vi "Measurement UI.vi"() -> ()   [LabVIEW 2023, in "FPT Pulse Measurement UI.lvlib"]
uses:
  FPT Pulse Measurement UI.lvlib
panel:
  in  "Measurement Graph":T1(tab)
  out "General Graph 1":T2(graph)
  out "General Graph 2":T2(graph)
  out "General Graph 3":T2(graph)
  in  "Power sequencing file validity check":bool
  out "TS Acquired Amplitude":dbl[][](array[numeric])
  out "Per Pulse Result (Name)":string[](array[string])
  out "Phase Stability (dB)":dbl
  out "Amplitude Stability (dB)":dbl
  out "Overshoot (%)":dbl
  out "Ripple (%)":dbl
  out "Droop (%)":dbl
  out "Fall Time (us)":dbl
  out "Rising Time (us)":dbl
  out "Duty Cycle (%)":dbl
  out "Per Pulse Result":dbl[][](array[numeric])
  in  "Power sequencing file path":string
  in  "RFSG name":string="5842_0"
  in  "RFSG attenuation mode":T3(ring)=enum."s2p File"
  in  "RFSG s2p file path":string
  in  "RFmx name":string="5842_0"
  in  "RFmx attenuation mode":T3(ring)=enum."s2p File"
  in  "RFmx s2p file path":string
  out "All graph references":refnum<vi>[](array[refnum])
  out "TS P2P Stability":dbl[][](array[numeric])
  out "TS Intrapulse Stability":dbl[][](array[numeric])
  out "MeasTable":string[][](table)
  out "MeasTable 2":string[][](table)
  in  "Configuration":T4(ring)
  in  "Tab Control":T5(tab)
  in  "Power sequencing file":path caption="Power Sequencing File Path"
  in  "RFmx port":string(combo)="port2" caption="RFmx Port"
  in  "RFSG port":string(combo)="port1" caption="RFSG Port"
  in  "RFSG name_update":refnum<k15> caption="RFSG Name"
  in  "RFSG attenuation mode_tab":T3(tab)=enum."s2p File" caption="RFSG Attenuation Mode"
  in  "RFSG external attenuation (dB)":dbl caption="External Attenuation" format="%#_6pdB"
  in  "RFSG s-parameters orientation":enum32{"Port1 Towards DUT", "Port2 Towards DUT"}(ring) caption="Orientation"
  in  "RFSG s2p file path_update":path caption="S2P File Path"
  in  "RFmx name_update":refnum<k15> caption="RFmx Name"
  in  "RFmx attenuation mode_tab":T3(tab)=enum."s2p File" caption="RFmx Attenuation Mode"
  in  "RFmx external attenuation (dB)":dbl caption="External Attenuation" format="%#_6pdB"
  in  "RFmx s-parameters orientation":enum32{"Port1 Towards DUT", "Port2 Towards DUT"}(ring) caption="Orientation"
  in  "RFmx s2p file path_update":path caption="S2P File Path"
  in  "RFmx Center Frequency (Hz)":dbl=10000000000.0 caption="Center Frequency" format="%#.3pHz"
  in  "RFmx Measurement Bandwidth (Hz)":dbl=80000000.0 caption="Measurement Bandwidth" format="%#.3pHz"
  in  "Pulse Acquisition Length (s)":dbl=0.001 caption="Pulse Acquisition Length" format="%#.3ps"
  in  "Pulse Power Level (dBm)":dbl=-20.0 caption="Pulse Power Level" format="%#.3pdBm"
  in  "Number of Pulses per Burst":u32=20
  in  "Pulse Width (s)":dbl=2e-05 caption="Pulse Width" format="%#.3ps"
  in  "Pulse Repetition Interval [PRI] (s)":dbl=0.0001 caption="Pulse Repetition Interval [PRI]" format="%#.3ps"
  in  "RFSG Generation IQ Rate (S/s)":dbl=1250000000.0 caption="Generation IQ Rate" format="%#.3pS/s"
  in  "RFmx Reference Level (dBm)":dbl=10.0 caption="Reference Level" format="%#.3pdBm"
  in  "Selected Pulse Trace":i32
  in  "Measurement Offset":i32
  in  "Window Step Size (%)":dbl=10.0 caption="Window Step Size" min=0.0 max=100.0 step=1.0 format="%#.3f%"
  in  "Window Stop (%)":dbl=90.0 caption="Window Stop" min=0.0 max=100.0 step=1.0 format="%d%"
  in  "Window Start (%)":dbl=10.0 caption="Window Start" min=0.0 max=100.0 step=1.0 format="%d%"
  in  "High Reference Level (%)":dbl=90.0 caption="High Reference Level" min=0.0 max=100.0 step=1.0 format="%d%"
  in  "Low Reference Level (%)":dbl=10.0 caption="Low Reference Level" min=0.0 max=100.0 step=1.0 format="%d%"
  in  "Width Reference Level (%)":dbl=50.0 caption="Width Reference Level" min=0.0 max=100.0 step=1.0 format="%d%"
  out "Status":string
  # "Pulse Stability"
  # "Pulse Profile"
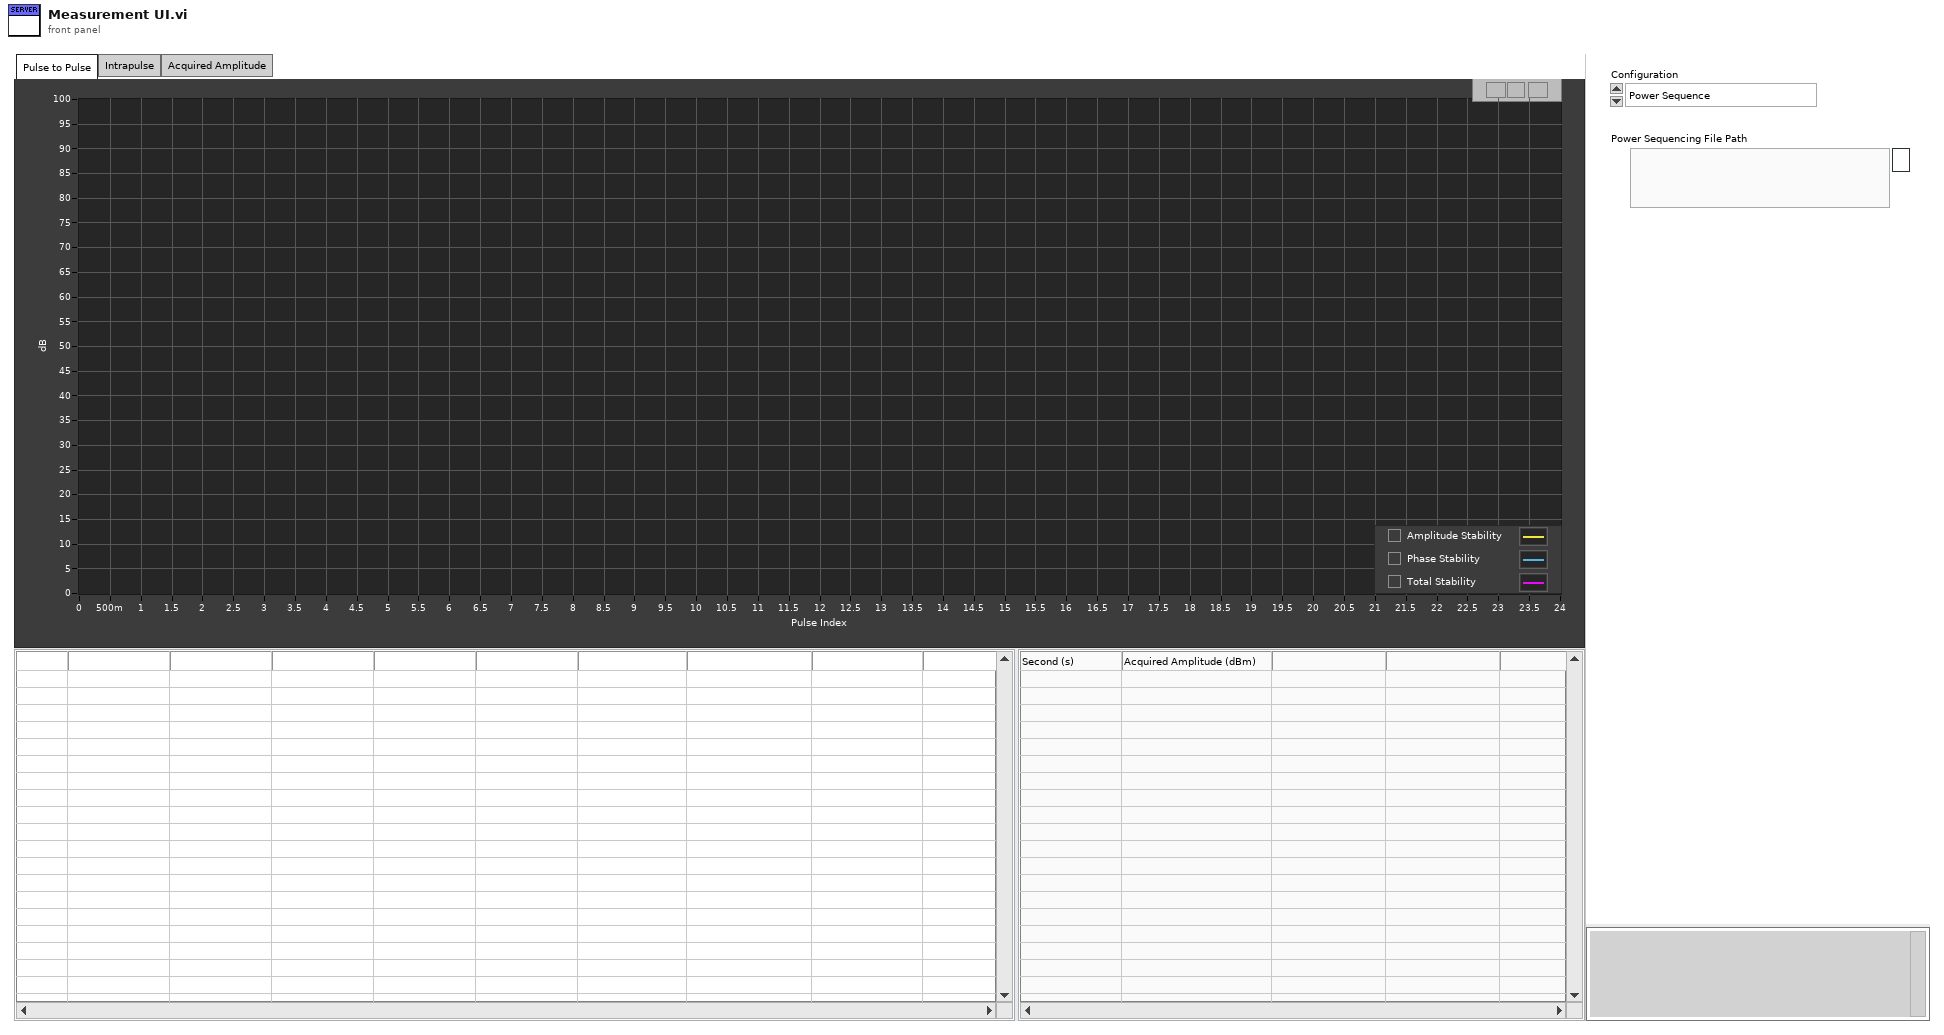
[diagram p1: front panel]
types:
  T1 = enum32{"Pulse to Pulse", "Intrapulse", "Acquired Amplitude", "Hidden Controls"}
  T2 = cluster{"Load currents":dbl[], "Efficiency":dbl[]}[]
  T3 = enum32{"<None>", "Constant Attenuation", "s2p File"}
  T4 = enum32{"Power Sequence", "HW + Correction", "Measurement 1", "Measurement 2"}
  T5 = enum32{"Power Sequence", "Correction", "Measurement 1", "Measurement 2"}
  T6 = cluster{"Shift":bool, "Ctrl":bool, "Alt":bool, "Cmd":bool, "Opt":bool}
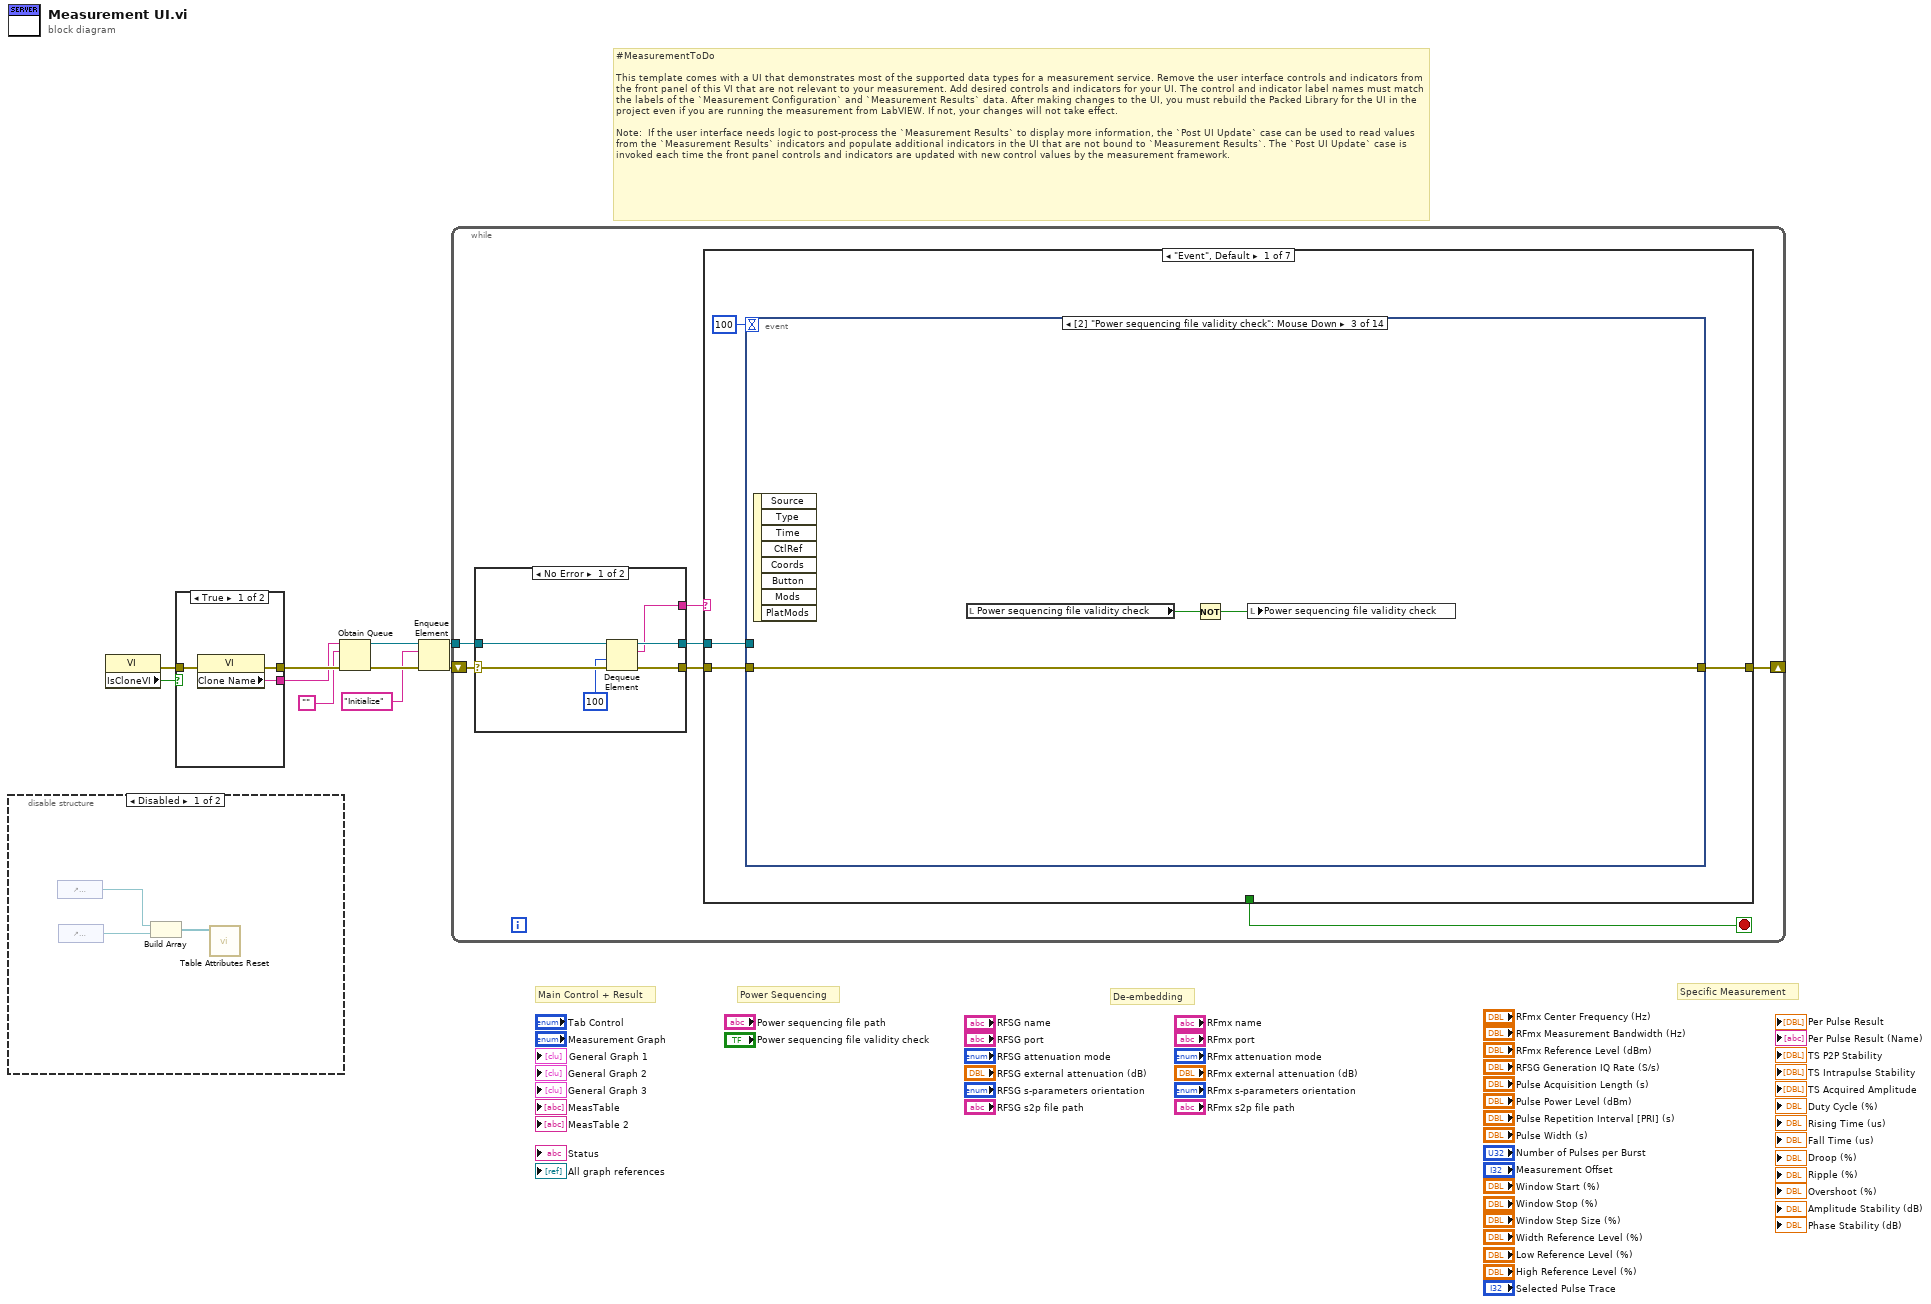
[diagram p0: block diagram]
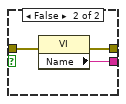
[diagram p3: hidden frame]
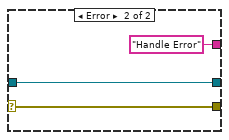
[diagram p4: hidden frame]
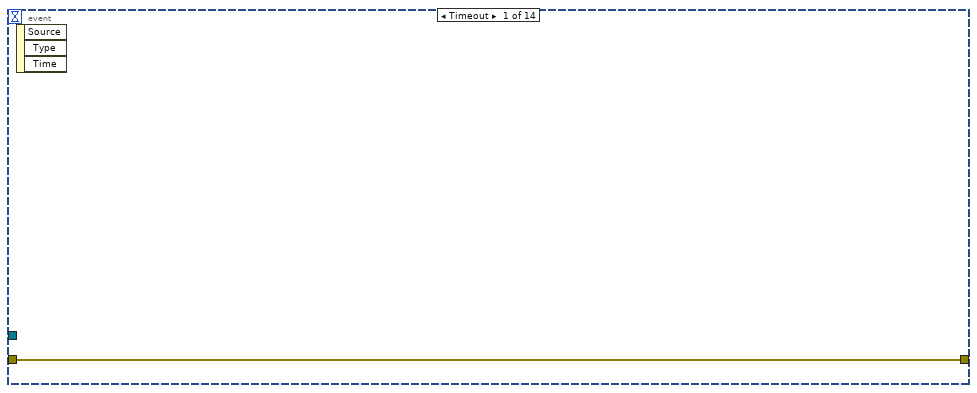
[diagram p5: hidden frame]
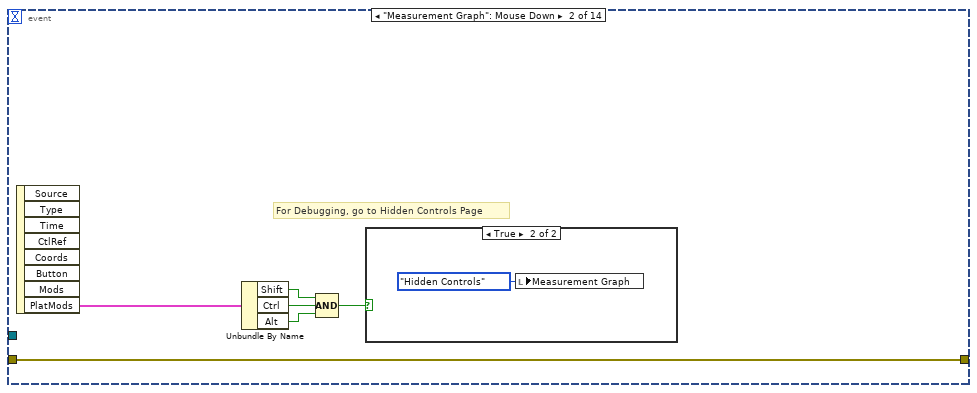
[diagram p6: hidden frame]
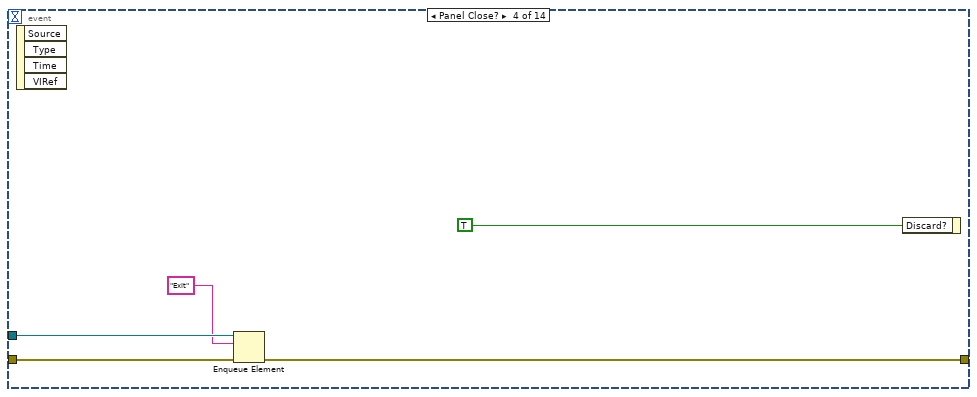
[diagram p8: hidden frame]
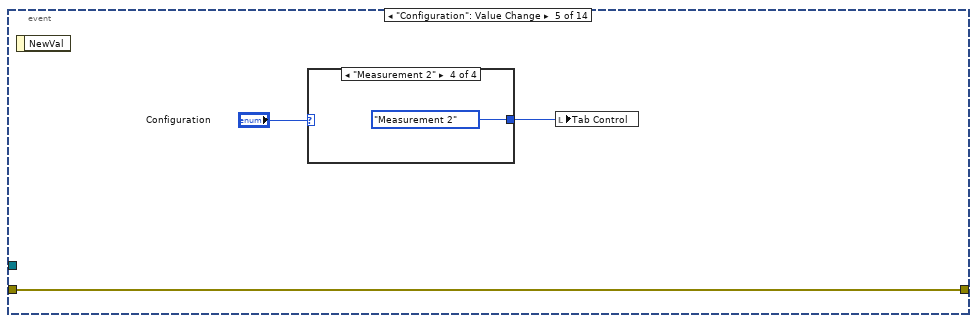
[diagram p9: hidden frame]
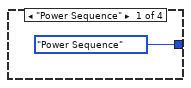
[diagram p10: hidden frame]
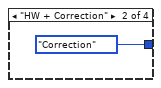
[diagram p11: hidden frame]
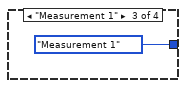
[diagram p12: hidden frame]
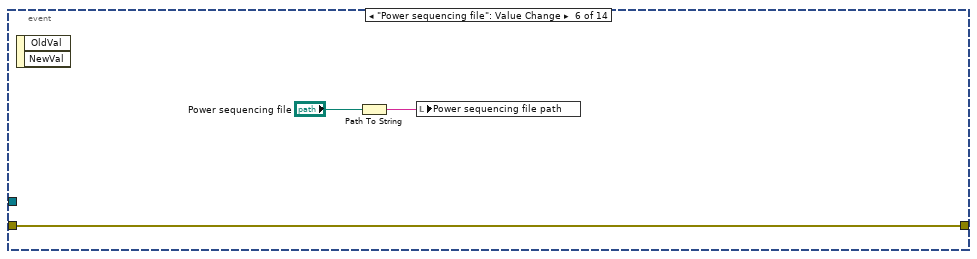
[diagram p13: hidden frame]
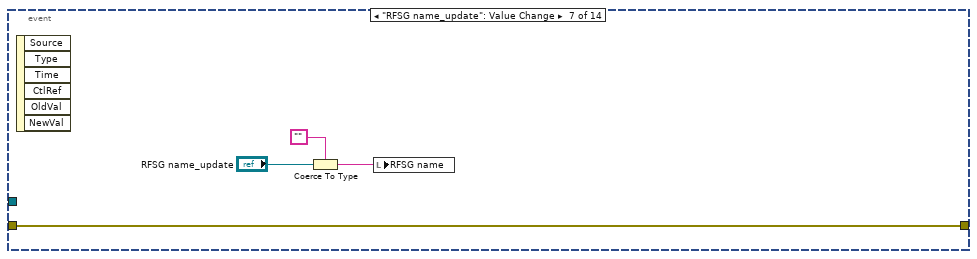
[diagram p14: hidden frame]
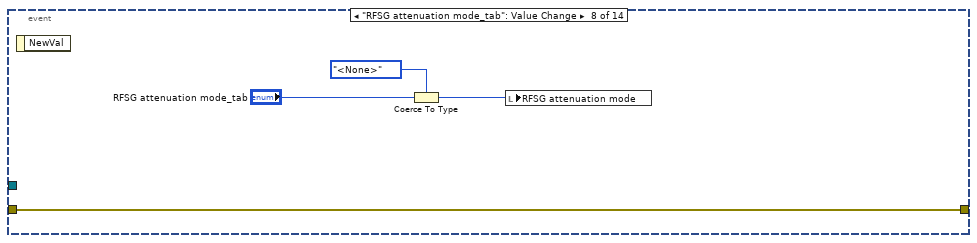
[diagram p15: hidden frame]
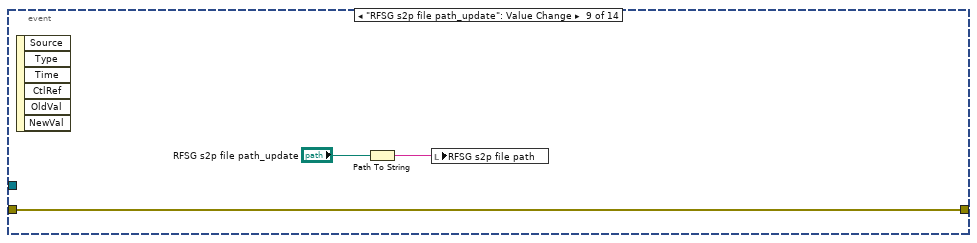
[diagram p16: hidden frame]
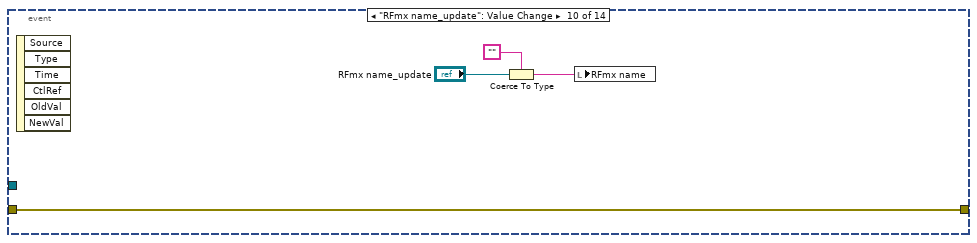
[diagram p17: hidden frame]
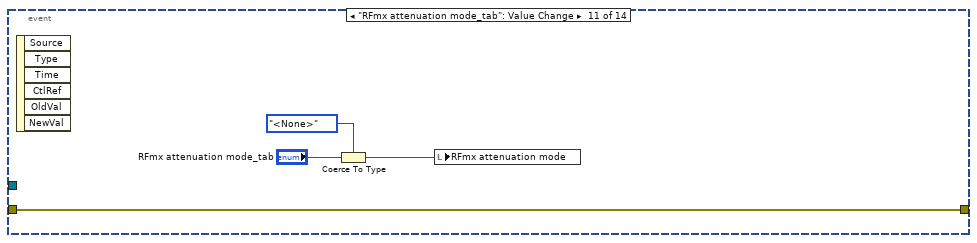
[diagram p18: hidden frame]
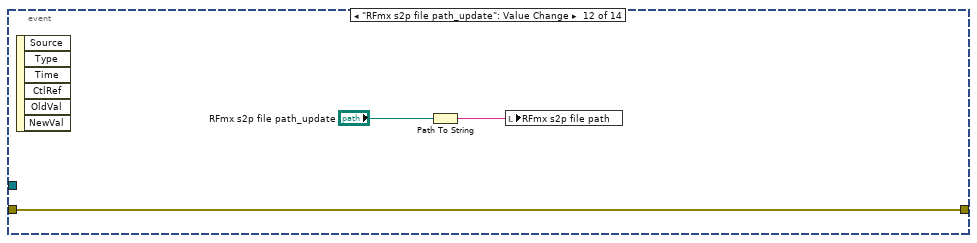
[diagram p19: hidden frame]
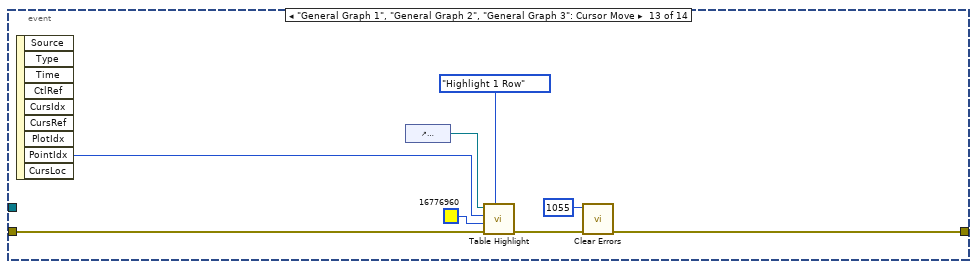
[diagram p20: hidden frame]
diagram:
  # "Specific Measurement"
  # "De-embedding"
  # "Power Sequencing"
  # "Main Control + Result"
  # "#MeasurementToDo  \n\nThis template comes with a UI that demonstrates most of the supported data types for a measurement service. Remove the user interface controls and indicators from the front panel of this VI that are not relevant to your measurement. Add desired controls and indicators for your UI. The control and indicator label names must match the labels of the `Measurement Configuration` and `Measurement Results` data. After making changes to the UI, you must rebuild the Packed Library for the UI in the project even if you are running the measurement from LabVIEW. If not, your changes will not take effect.\n\nNote:  If the user interface needs logic to post-process the `Measurement Results` to display more information, the `Post UI Update` case can be used to read values from the `Measurement Results` indicators and populate additional indicators in the UI that are not bound to `Measurement Results`. The `Post UI Update` case is invoked each time the front panel controls and indicators are updated with new control values by the measurement framework."
  n1 = disable-structure shown="Disabled" {
    frame Disabled {
      n2 = control-ref of="MeasTable"() -> (w12:refnum<vi>)
      n3 = control-ref of="MeasTable 2"() -> (w13:refnum<vi>)
      n4 = Build Array(w12, w13) -> (w11:refnum<vi>[])
      n5 = call "Table Attributes Reset.vi"("Table Refs"=w11) -> ()  [unwired: 11 in]
    }
    frame Enabled {
    }
  }
  n6 = property class="VI"() -> (error out=w1:errorcluster, "IsCloneVI"=w2:bool)  [unwired: 2 in, 1 out]
  n7 = case shown="True" w2 {
    tunnel: [w16 w19] -> w10
    tunnel: [w15 w18] -> w9
    tunnel: w1 -> [w14 w17]
    frame True {
      n8 = property class="VI"(error in=w14) -> (error out=w16:errorcluster, "Clone Name"=w15:string)  [unwired: 1 in, 1 out]
    }
    frame False {
      n9 = property class="VI"(error in=w17) -> (error out=w19:errorcluster, "Name"=w18:string)  [unwired: 1 in, 1 out]
    }
  }
  n10 = Obtain Queue(name (unnamed)=w9, element data type="", error in (no error)=w10) -> (queue out=w6:refnum<queue>, error out=w8:errorcluster)  [unwired: 2 in, 1 out]
  n11 = Enqueue Element(queue=w6, element="Initialize", error in (no error)=w8) -> (queue out=w5:refnum<queue>, error out=w7:errorcluster)  [unwired: 1 in, 1 out]
  n12 = while {
    shift-right: [w21] -> _
    shift-left: w7 -> [w26]
    tunnel: w5 -> [w24]
    stop <- w20 stop-if-true
    n13 = case shown="No Error" w26 {
      selector: w26 -> [w32 w35]
      tunnel: [w31 w35] -> w25
      tunnel: w24 -> [w30 w34]
      tunnel: [w29 w34] -> w23
      tunnel: [w28 "Handle Error"] -> w22
      frame No Error {
        n14 = Dequeue Element(queue=w30, timeout in ms (-1)=100, error in (no error)=w32) -> (queue out=w29:refnum<queue>, element=w28:string, error out=w31:errorcluster)  [unwired: 1 out]
      }
      frame Error {
      }
    }
    n15 = case shown="\"Event\", Default" w22 {
      tunnel: w25 -> [w38 w132 w153 w202 w220 w227 w228]
      tunnel: w23 -> [w36 _ w152 w201 _ w225 _]
      tunnel: [w39 w132 w153 w179 w216 w222 w228] -> w21
      tunnel: [_ _ _ _ _ TRUE _] -> w20
      frame "Event", Default {
        n16 = event shown="[2] \"Power sequencing file validity check\": Mouse Down" {
          selector: _ -> [_ _ _ _ _ _ _ _ _ _ _ _ _ _]
          dyn-events: _ -> [_ _ _ _ _ _ _ _ _ _ _ _ _ _]
          timeout: 100 -> [_ _ _ _ _ _ _ _ _ _ _ _ _ _]
          tunnel: [w40 w41 w48 w53 w56 w63 w66 w70 w74 w77 w81 w85 w90 w106] -> w39
          tunnel: w38 -> [w40 w41 w48 w54 w56 w63 w66 w70 w74 w77 w81 w85 w88 w105]
          tunnel: w36 -> [_ _ _ w52 _ _ _ _ _ _ _ _ _ _]
          event Timeout {
            n17 = event-data() -> ()  [unwired: 1 in, 3 out]
          }
          event "Measurement Graph": Mouse Down {
            # "For Debugging, go to Hidden Controls Page"
            n18 = event-data() -> ("PlatMods"=w42:T6)  [unwired: 1 in, 7 out]
            n19 = Unbundle By Name(w42) -> ("Shift"=w46:bool, "Ctrl"=w45:bool, "Alt"=w44:bool)
            n20 = Compound Arithmetic op=AND(w46, w45, w44) -> (w43:bool)
            n21 = case shown="True" w43 {
              frame False {
              }
              frame True {
                n22 = local write "Measurement Graph"(T1."Hidden Controls" ("Measurement Graph")) -> ()
              }
            }
          }
          event "Power sequencing file validity check": Mouse Down {
            n23 = event-data() -> ()  [unwired: 1 in, 8 out]
            n24 = local read "Power sequencing file validity check"() -> (w50:bool)
            n25 = Not(x=w50) -> (.not. x?=w49:bool)
            n26 = local write "Power sequencing file validity check"(w49) -> ()
          }
          event Panel Close? {
            n27 = event-data() -> ()  [unwired: 1 in, 4 out]
            n28 = Enqueue Element(queue=w52, element="Exit", error in (no error)=w54) -> (error out=w53:errorcluster)  [unwired: 1 in, 2 out]
            n29 = event-data("Discard?"=TRUE) -> ()  [unwired: 1 in, 1 out]
          }
          event "Configuration": Value Change {
            n30 = event-data() -> ()  [unwired: 1 in, 1 out]
            n31 = case shown="\"Measurement 2\"" "Configuration" {
              tunnel: [T5."Power Sequence" ("Tab Control") T5."Correction" ("Tab Control") T5."Measurement 1" ("Tab Control") T5."Measurement 2" ("Tab Control")] -> w57
              frame "Power Sequence" {
              }
              frame "HW + Correction" {
              }
              frame "Measurement 1" {
              }
              frame "Measurement 2" {
              }
            }
            n32 = local write "Tab Control"(w57) -> ()
          }
          event "Power sequencing file": Value Change {
            n33 = event-data() -> ()  [unwired: 1 in, 2 out]
            n34 = Path To String(path="Power sequencing file") -> (string=w64:string)
            n35 = local write "Power sequencing file path"(w64) -> ()
          }
          event "RFSG name_update": Value Change {
            n36 = event-data() -> ()  [unwired: 1 in, 6 out]
            n37 = Coerce To Type(0:"RFSG name_update", 1:"") -> (2:w67:string)
            n38 = local write "RFSG name"(w67) -> ()
          }
          event "RFSG attenuation mode_tab": Value Change {
            n39 = event-data() -> ()  [unwired: 1 in, 1 out]
            n40 = Coerce To Type(0:"RFSG attenuation mode_tab", 1:T3."<None>" ("RFSG attenuation mode")) -> (2:w73:T3)
            n41 = local write "RFSG attenuation mode"(w73) -> ()
          }
          event "RFSG s2p file path_update": Value Change {
            n42 = event-data() -> ()  [unwired: 1 in, 6 out]
            n43 = Path To String(path="RFSG s2p file path_update") -> (string=w75:string)
            n44 = local write "RFSG s2p file path"(w75) -> ()
          }
          event "RFmx name_update": Value Change {
            n45 = event-data() -> ()  [unwired: 1 in, 6 out]
            n46 = Coerce To Type(0:"RFmx name_update", 1:"") -> (2:w79:string)
            n47 = local write "RFmx name"(w79) -> ()
          }
          event "RFmx attenuation mode_tab": Value Change {
            n48 = event-data() -> ()  [unwired: 1 in, 6 out]
            n49 = Coerce To Type(0:"RFmx attenuation mode_tab", 1:T3."<None>" ("RFmx attenuation mode")) -> (2:w83:T3)
            n50 = local write "RFmx attenuation mode"(w83) -> ()
          }
          event "RFmx s2p file path_update": Value Change {
            n51 = event-data() -> ()  [unwired: 1 in, 6 out]
            n52 = Path To String(path="RFmx s2p file path_update") -> (string=w86:string)
            n53 = local write "RFmx s2p file path"(w86) -> ()
          }
          event "General Graph 1", "General Graph 2", "General Graph 3": Cursor Move {
            n54 = event-data() -> ("PointIdx"=w95:i32)  [unwired: 1 in, 8 out]
            n55 = control-ref of="MeasTable 2"() -> (w93:refnum<vi>)
            n56 = call "Table Highlight.vi"("Action"=enum16{"Reset", "Highlight 1 Row"}."Highlight 1 Row", "error in"=w88, "Color Box"=u32 16776960, "Row"=w95, "Table Ref in"=w93) -> ("error out"=w91:errorcluster)  [unwired: 5 in, 1 out]
            n57 = call <vilib>:"Clear Errors.vi"("error in (no error)"=w91, "specific error code to clear (0: all)"=1055) -> ("error out"=w90:errorcluster)  [unwired: 4 in, 1 out]
          }
          event "Measurement Graph": Value Change {
            n58 = event-data() -> ("NewVal"=w101:T1)  [unwired: 1 in, 5 out]
            n59 = local read "TS Acquired Amplitude"() -> (w97:dbl[][])
            n60 = local read "TS Intrapulse Stability"() -> (w99:dbl[][])
            n61 = local read "TS P2P Stability"() -> (w100:dbl[][])
            n62 = case shown="\"Acquired Amplitude\"" w101 {
              tunnel: [w123 w124 w125] -> w103
              frame "Pulse to Pulse", Default {
                n63 = control-ref of="General Graph 1"() -> (w123:refnum<vi>)
              }
              frame "Intrapulse" {
                n64 = control-ref of="General Graph 2"() -> (w124:refnum<vi>)
              }
              frame "Acquired Amplitude" {
                n65 = control-ref of="General Graph 3"() -> (w125:refnum<vi>)
              }
            }
            n66 = case shown="\"Pulse to Pulse\", Default" w101 {
              tunnel: w99 -> [_ w118 _]
              tunnel: w100 -> [w114 _ _]
              tunnel: [w114 w118 w119] -> w98
              tunnel: w97 -> [_ _ w119]
              tunnel: [w111 w115 w120] -> w96
              frame "Pulse to Pulse", Default {
                n67 = Build Array (concatenate)("Pulse Index", string[] ["Amplitude Stability (dB)", "Phase Stability (dB)", "Total Stability (dB)"]) -> (w111:string[])
              }
              frame "Intrapulse" {
                n68 = Build Array (concatenate)("Second (s)", string[] ["Amplitude Stability (dB)", "Phase Stability (dB)", "Total Stability (dB)"]) -> (w115:string[])
              }
              frame "Acquired Amplitude" {
                n69 = Build Array (concatenate)("Second (s)", string[] ["Acquired Amplitude (dBm)"]) -> (w120:string[])
              }
            }
            n70 = Build Array(w103) -> (w102:refnum<vi>[])
            n71 = call "Graph Cursor Update.vi"("Action"=enum16{"Reset", "Update"}."Reset", "error in"=w105, "Cursor Type"=enum16{"Movable", "Fixed", "All"}."Movable", "Graph Refs in"=w102) -> ("error out"=w107:errorcluster)  [unwired: 6 in, 1 out]
            n72 = control-ref of="MeasTable 2"() -> (w104:refnum<vi>)
            n73 = call "Table Set Header Name and Data (DBL).vi"("Data"=w98, "Header"=w96, "Table Ref"=w104) -> ()  [unwired: 9 in]
            n74 = call "Table Highlight.vi"("Action"=enum16{"Reset", "Highlight 1 Row"}."Reset", "error in"=w107, "Table Ref in"=w104) -> ("error out"=w106:errorcluster)  [unwired: 7 in, 1 out]
          }
        }
      }
      frame "Initialize" {
        w131 = 0
        n75 = control-ref of="General Graph 1"() -> (w130:refnum<vi>)
        n76 = control-ref of="General Graph 2"() -> (w129:refnum<vi>)
        n77 = control-ref of="General Graph 3"() -> (w126:refnum<vi>)
        n78 = Build Array(w130, w129, w126) -> (w127:refnum<vi>[])
        n79 = local write "Tab Control"(w131) -> ()
        n80 = local write "Configuration"(w131) -> ()
        n81 = local write "All graph references"(w127) -> ()
        n82 = call "Graph Set Cursor Mode.vi"("Cursor Mode"=enum32{"Free-Drag", "Single-Plot", "Multi-Plot"}."Multi-Plot", "Graph Refs in"=w127) -> ()  [unwired: 8 in, 2 out]
      }
      frame "Post UI Update" {
        # "This case will be triggered, after framework updates the User interface with result values.\nUsed to update data type def"
        n83 = local read "Power sequencing file path"() -> (w149:string)
        n84 = local read "RFSG name"() -> (w146:string)
        n85 = local read "RFSG attenuation mode"() -> (w148:T3)
        n86 = local read "RFSG s2p file path"() -> (w142:string)
        n87 = Coerce To Type(0:w146, 1:refnum<k15> refnum ("RFSG name_update")) -> (2:w144:refnum<k15>)
        n88 = Enqueue Element(queue=w152, element="Post UI Update 2") -> ()  [unwired: 2 in, 3 out]
        n89 = local write "RFSG name_update"(w144) -> ()
        n90 = Coerce To Type(0:w148, 1:T3."<None>" ("RFSG attenuation mode_tab")) -> (2:w147:T3)
        n91 = String To Path(string=w149) -> (path=w150:path)
        n92 = String To Path(string=w142) -> (path=w143:path)
        n93 = local write "RFSG attenuation mode_tab"(w147) -> ()
        n94 = local write "RFSG s2p file path_update"(w143) -> ()
        n95 = local write "Power sequencing file"(w150) -> ()
        n96 = local read "RFmx name"() -> (w137:string)
        n97 = local read "RFmx attenuation mode"() -> (w135:T3)
        n98 = local read "RFmx s2p file path"() -> (w141:string)
        n99 = Coerce To Type(0:w137, 1:refnum<k15> refnum ("RFSG name_update")) -> (2:w139:refnum<k15>)
        n100 = local write "RFmx name_update"(w139) -> ()
        n101 = Coerce To Type(0:w135, 1:T3."<None>" ("RFmx attenuation mode_tab")) -> (2:w136:T3)
        n102 = String To Path(string=w141) -> (path=w140:path)
        n103 = local write "RFmx attenuation mode_tab"(w136) -> ()
        n104 = local write "RFmx s2p file path_update"(w140) -> ()
      }
      frame "Post UI Update 2" {
        # "Run after Post UI Update. Can be duplicate is need more processing.\nUtilize this case to convert the result to graph or table"
        n105 = local read "TS Acquired Amplitude"() -> (w154:dbl[][])
        n106 = local read "TS Intrapulse Stability"() -> (w158:dbl[][])
        n107 = local read "TS P2P Stability"() -> (w159:dbl[][])
        n108 = local read "Measurement Graph"() -> (w160:T1)
        n109 = Enqueue Element(queue=w201, element="Post UI Update 3", error in (no error)=w202) -> (error out=w180:errorcluster)  [unwired: 1 in, 2 out]
        n110 = local read "Amplitude Stability (dB)"() -> (w196:dbl)
        n111 = local read "Phase Stability (dB)"() -> (w197:dbl)
        n112 = local read "Rising Time (us)"() -> (w191:dbl)
        n113 = local read "Overshoot (%)"() -> (w195:dbl)
        n114 = local read "Duty Cycle (%)"() -> (w190:dbl)
        n115 = local read "Fall Time (us)"() -> (w192:dbl)
        n116 = local read "Per Pulse Result"() -> (w171:dbl[][])
        n117 = local read "Droop (%)"() -> (w193:dbl)
        n118 = local read "Ripple (%)"() -> (w194:dbl)
        n119 = case shown="\"Pulse to Pulse\", Default" w160 {
          tunnel: w158 -> [_ w211 _]
          tunnel: w159 -> [w207 _ _]
          tunnel: [w207 w211 w213] -> w162
          tunnel: w154 -> [_ _ w213]
          tunnel: [w205 w209 w214] -> w161
          tunnel: [w204 w208 w212] -> w156
          frame "Pulse to Pulse", Default {
            w204 = string[] ["Amplitude Stability (dB)", "Phase Stability (dB)", "Total Stability (dB)"]
            n120 = Build Array (concatenate)("Pulse Index", w204) -> (w205:string[])
          }
          frame "Intrapulse" {
            w208 = string[] ["Amplitude Stability (dB)", "Phase Stability (dB)", "Total Stability (dB)"]
            n121 = Build Array (concatenate)("Second (s)", w208) -> (w209:string[])
          }
          frame "Acquired Amplitude" {
            w212 = string[] ["Acquired Amplitude (dBm)"]
            n122 = Build Array (concatenate)("Second (s)", w212) -> (w214:string[])
          }
        }
        n123 = Build Array(w190, w191, w192, w193, w194, w195, w196, w197) -> (w189:dbl[])
        n124 = Delete From Array(array=w171, index (row)=0) -> (deleted portion=w167:dbl[], array with subset deleted=w169:dbl[][])  [unwired: 2 in]
        n125 = Number To Fractional String(number=w189) -> (F-format string=w188:string[])  [unwired: 3 in]
        n126 = Number To Fractional String(number=w169) -> (F-format string=w165:string[][])  [unwired: 3 in]
        n127 = Number To Fractional String(number=w167, precision (6)=i16 0) -> (F-format string=w166:string[])  [unwired: 2 in]
        n128 = Insert Into Array(array=w188, index=0, new element="Average" ("new element/subarray")) -> (w184:string[])
        n129 = Build Array (concatenate)(w166, w165) -> (w164:string[][])
        n130 = Transpose 2D Array(2D array=w164) -> (transposed array=w163:string[][])
        n131 = Build Array (concatenate)(w163, w184) -> (w174:string[][])
        n132 = control-ref of="MeasTable 2"() -> (w198:refnum<vi>)
        n133 = Transpose 2D Array(2D array=w174) -> (transposed array=w176:string[][])
        n134 = Array Size(array=w174) -> (size(s)=w175:i32[])
        n135 = local read "Per Pulse Result (Name)"() -> (w183:string[])
        n136 = control-ref of="General Graph 1"() -> (w200:refnum<vi>)
        n137 = control-ref of="General Graph 2"() -> (w199:refnum<vi>)
        n138 = control-ref of="General Graph 3"() -> (w155:refnum<vi>)
        n139 = call "Table Set Header Name and Data (DBL).vi"("Data"=w162, "Header"=w161, "Table Ref"=w198) -> ()  [unwired: 9 in]
        n140 = Index Array(array=w175) -> (element=w173:i32)  [unwired: 1 in]
        n141 = Decrement(x=w173) -> (x-1=w172:i32)
        n142 = control-ref of="MeasTable"() -> (w185:refnum<vi>)
        n143 = call "Graph Assign Plot Names and Data.vi"("Legend Number of Rows"=3, "X Ys Data"=w159, "Plot Names"=w156, "Graph Ref in"=w200) -> ()  [unwired: 5 in, 3 out]
        n144 = call "Graph Assign Plot Names and Data.vi"("Legend Number of Rows"=3, "X Ys Data"=w158, "Plot Names"=w156, "Graph Ref in"=w199) -> ()  [unwired: 5 in, 3 out]
        n145 = call "Graph Assign Plot Names and Data.vi"("Legend Number of Rows"=1, "X Ys Data"=w154, "Plot Names"=w156, "Graph Ref in"=w155) -> ()  [unwired: 5 in, 3 out]
        n146 = call "Table Set Header Name and Data (String).vi"("Data"=w176, "Header"=w183, "Table Ref"=w185) -> ()  [unwired: 9 in]
        n147 = control-ref of="MeasTable"() -> (w178:refnum<vi>)
        n148 = call "Table Highlight.vi"("Action"=enum16{"Reset", "Highlight 1 Row"}."Highlight 1 Row", "error in"=w180, "Row"=w172, "Table Ref in"=w178) -> ("error out"=w179:errorcluster)  [unwired: 6 in, 1 out]
      }
      frame "Post UI Update 3" {
        n149 = local read "All graph references"() -> (w219:refnum<vi>[])
        n150 = call "Graph Cursor Update.vi"("Action"=enum16{"Reset", "Update"}."Reset", "error in"=w220, "Cursor Type"=enum16{"Movable", "Fixed", "All"}."Movable", "Graph Refs in"=w219) -> ("error out"=w216:errorcluster)  [unwired: 6 in, 1 out]
      }
      frame "Exit" {
        # "This case is triggered to close the User Interface from framework"
        n151 = Flush Queue(queue=w225, error in (no error)=w227) -> (queue out=w224:refnum<queue>, error out=w223:errorcluster)  [unwired: 1 out]
        n152 = Release Queue(queue=w224, force destroy? (F)=TRUE, error in (no error)=w223) -> (error out=w222:errorcluster)  [unwired: 2 out]
      }
      frame "Handle Error" {
      }
    }
  }
